vi "Untitled 4.vi"() -> ()   [LabVIEW 2020]
panel:
  in  "Discharge Stop Voltage(V) 2":dbl
  in  "Discharge Current(A)":dbl
  in  "Discharge Voltage(V)":dbl
  in  "Charge Current(A)":dbl
  in  "Charge Voltage(V)":dbl
  in  "VISA resource name":refnum<visa-resource-name>
  in  "Charge Stop Voltage(V)":dbl
  in  "stop":bool
  out "Read Current(A)":dbl format="%.2g"
  out "Read Voltage(V)":dbl format="%.2g"
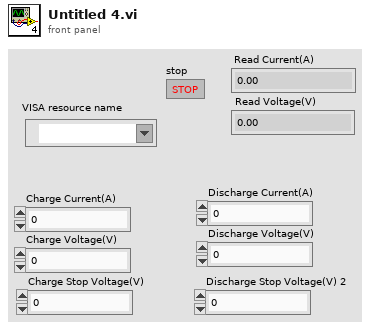
[diagram p1: front panel]
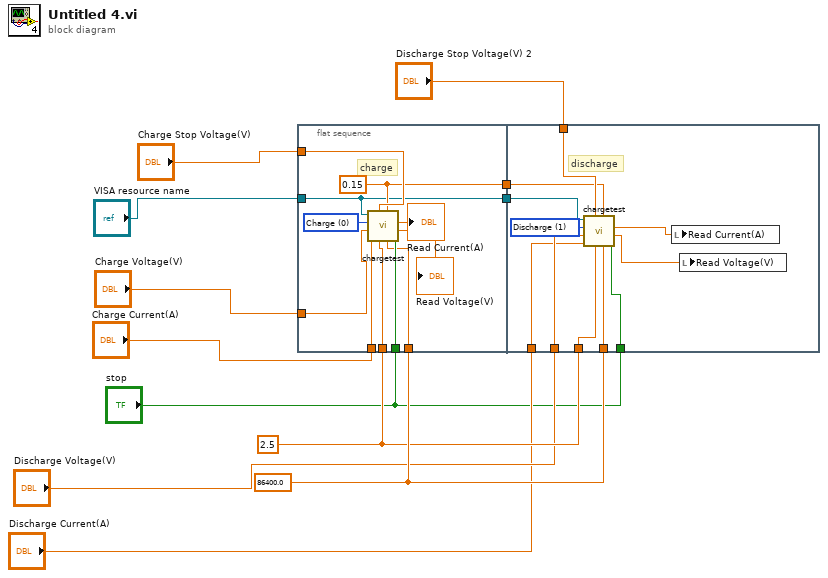
[diagram p0: block diagram]
diagram:
  w5 = 2.5 ("Stop Capacity(Ah)")
  w6 = 86400.0 ("Stop Time(s)")
  n1 = flat-sequence {
    tunnel: "Charge Stop Voltage(V)" -> [w23]
    tunnel: "VISA resource name" -> [w13]
    tunnel: "Charge Voltage(V)" -> [w22]
    tunnel: "Charge Current(A)" -> [w21]
    tunnel: "stop" -> [w20]
    tunnel: w6 -> [w19]
    tunnel: w5 -> [w18]
    tunnel: [w14] -> w12
    tunnel: [w13] -> w11
    tunnel: w6 -> [w34]
    tunnel: w5 -> [w33]
    tunnel: "Discharge Voltage(V)" -> [w32]
    tunnel: "Discharge Current(A)" -> [w31]
    tunnel: "stop" -> [w27]
    tunnel: "Discharge Stop Voltage(V) 2" -> [w26]
    tunnel: w12 -> [w25]
    tunnel: w11 -> [w24]
    frame #0 {
      w14 = 0.15 ("Stop Current(A)")
      w17 = u8 0 items=["Charge", "Discharge"] ("Battery Mode")
      # "charge"
      n2 = call <instrlib>:"chargetest.vi"("stop"=w20, "Stop Time(s)"=w19, "Stop Current(A)"=w14, "Stop Capacity(Ah)"=w18, "Stop Voltage(V)"=w23, "Charge\\Discharge Current(A)"=w21, "Charge\\Discharge Voltage(V)"=w22, "Battery Mode"=w17, "VISA resource name"=w13) -> ("Read Voltage(V)"=→"Read Voltage(V)":dbl, "Read Current(A)"=→"Read Current(A)":dbl)  [unwired: 1 in]
    }
    frame #1 {
      w30 = u8 1 items=["Charge", "Discharge"] ("Battery Mode")
      # "discharge"
      n3 = call <instrlib>:"chargetest.vi"("stop"=w27, "Stop Time(s)"=w34, "Stop Current(A)"=w25, "Stop Capacity(Ah)"=w33, "Stop Voltage(V)"=w26, "Charge\\Discharge Current(A)"=w31, "Charge\\Discharge Voltage(V)"=w32, "Battery Mode"=w30, "VISA resource name"=w24) -> ("Read Voltage(V)"=w28:dbl, "Read Current(A)"=w29:dbl)  [unwired: 1 in]
      n4 = local write "Read Current(A)"(w29) -> ()
      n5 = local write "Read Voltage(V)"(w28) -> ()
    }
  }
